vi "SortByNumber.vi"(8 "error in (no error)":errorcluster, 10 "Sort by":string, 11 "Products":T1[](array[typedef])) -> (0 "error out":errorcluster, 3 "Sorted Products":T1[](array[typedef]))   [LabVIEW 2022 SP3]
uses:
  e174fcb8-0b4a-4fb4-bd9f-c3c7b4d6588e.vi
  #typedef_product.ctl
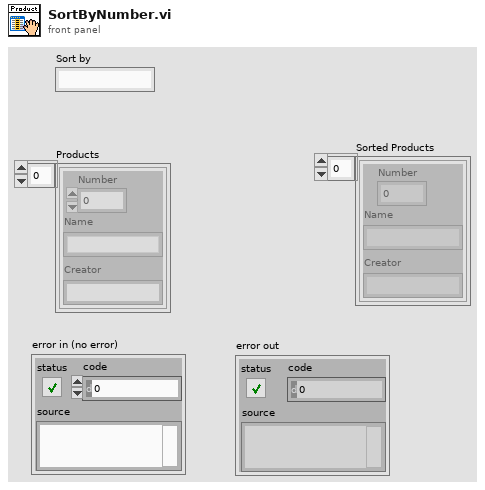
[diagram p1: front panel]
types:
  T1 = typedef "#typedef_product.ctl" = cluster{"Number ":i32, "Name":string, "Creator":string}
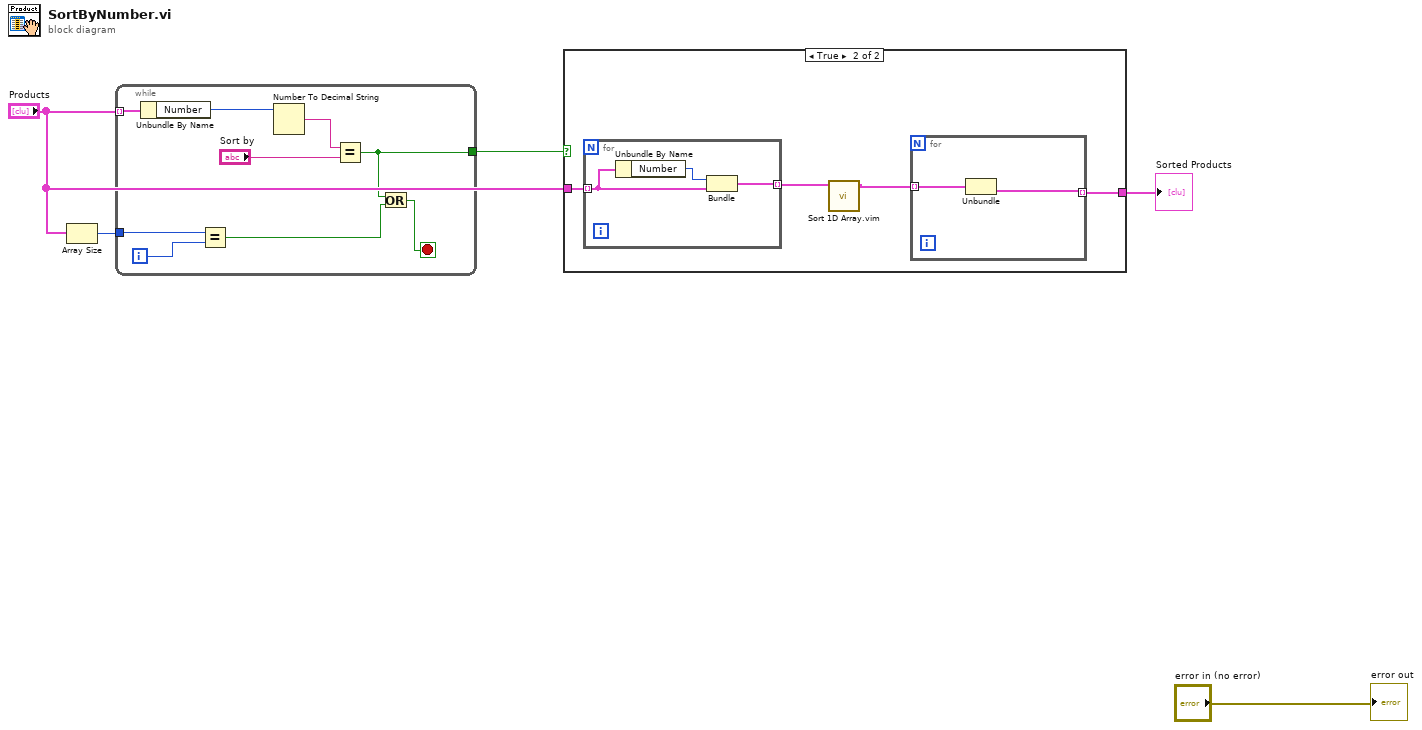
[diagram p0: block diagram]
diagram:
  n1 = Array Size(array="Products") -> (size(s)=w3:i32)
  n2 = while {
    tunnel: "Products" -> [w11] mode=indexing
    tunnel: w3 -> [w10]
    tunnel: [w6] -> w2
    i -> [w9]
    stop <- w7 stop-if-true
    n3 = Unbundle By Name(w11) -> ("Number"=w14:i32)
    n4 = Equal?(x=w10, y=w9) -> (x = y?=w8:bool)
    n5 = Number To Decimal String(number=w14) -> (decimal integer string=w13:string)  [unwired: 1 in]
    n6 = Equal?(x=w13, y="Sort by") -> (x = y?=w6:bool)
    n7 = Or(x=w6, y=w8) -> (x .or. y?=w7:bool)
  }
  n8 = case shown="True" w2 {
    tunnel: [w15 w17] -> w1
    tunnel: "Products" -> [w15 w16]
    frame False {
    }
    frame True {
      n9 = for {
        tunnel: w16 -> [w23] mode=indexing
        tunnel: [w22] -> w19 mode=indexing
        n10 = Unbundle By Name(w23) -> ("Number"=w24:i32)
        n11 = Bundle("Number"=w24, "Product"=w23) -> (w22:cluster{"Number ":i32, "Product":T1})  [unwired: 1 in]
      }
      n12 = call "Sort 1D Array.vim"("unsorted array"=w19) -> ("sorted array"=w18:cluster{"Number ":i32, "Product":T1}[])  [unwired: 10 in]
      n13 = for {
        tunnel: w18 -> [w21] mode=indexing
        tunnel: [w20] -> w17 mode=indexing
        n14 = Unbundle(w21) -> ("Product"=w20:T1)  [unwired: 1 out]
      }
    }
  }
  "Sorted Products" <- w1
  "error out" <- "error in (no error)"
